vi "Test Parse Date String.vi"(8 "error in (no error)":errorcluster, 11 "Test Case In":refnum<class "Barcode Test.lvclass">) -> (0 "error out":errorcluster, 3 "Test Case Out":refnum<class "Barcode Test.lvclass">)   [LabVIEW 2020, in "Barcode Reader First Iteration.lvlib" / "Barcode Test.lvclass"]
uses:
  Barcode Test.lvclass
  Barcode Test.lvclass/Barcode Test.ctl
  01074fa8-ee8a-411d-bc8b-fc92c4f90959.vi
  Barcode Reader/Barcode.lvclass
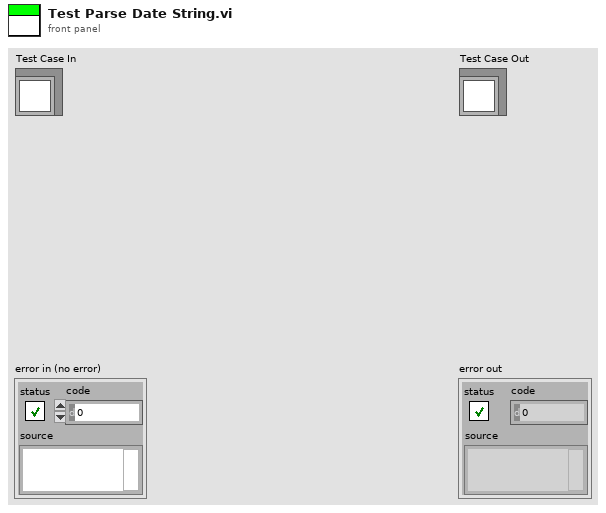
[diagram p1: front panel]
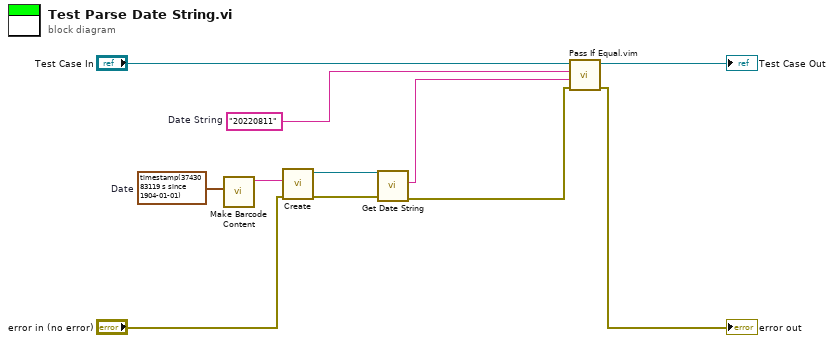
[diagram p0: block diagram]
diagram:
  w1 = "20220811"  # Date String
  w2 = timestamp(3743083119.3780074 s since 1904-01-01)  # Date
  n1 = call "Make Barcode Content.vi"("Date"=w2) -> ("Barcode Content"=w8:string)  [unwired: 10 in]
  n2 = call "Create.vi"("error in (no error)"="error in (no error)", "Barcode Content"=w8) -> ("error out"=w5:errorcluster, "Barcode Reader out"=w7:refnum<class "Barcode.lvclass">)  [unwired: 8 in]
  n3 = call "Get Date String.vi"("error in (no error)"=w5, "Barcode Reader in"=w7) -> ("error out"=w3:errorcluster, "Serial Number"=w6:string)  [unwired: 7 in, 1 out]
  n4 = call "Pass If Equal.vim"("error in (no error)"=w3, "Actual"=w6, "Expected"=w1, "LUnit Test Case In"="Test Case In") -> ("error out"=→"error out":errorcluster, "LUnit Test Case Out"=→"Test Case Out":refnum<class "Barcode Test.lvclass">)  [unwired: 6 in]
